vi "SMO.Control Experiment.getKHShuntType.vi"(8 "error in (no error)":errorcluster, 10 "getKHShuntType":T1, 11 "Control Experiment":refnum<class "SMO.Control Experiment.lvclass">) -> (0 "error out":errorcluster, 3 "Control Experiment out":refnum<class "SMO.Control Experiment.lvclass">)   [LabVIEW 2019, in "SMO.Control Experiment.lvclass"]
doc: "---------------------------------------------------------------\nJKI State Machine Objects™\nhttp://jki.net/state-machine-objects/\nCopyright (C) 2005-2015, JKI <info@jki.net>\nALL RIGHTS RESERVEDJKI State Machine Objects (SMO) 1.0.0.4\nJKI - JKI\nCopyright (c) 2015, JKI"
uses:
  SMO.Control Experiment.lvclass
  Typedefs/PublicEvents--SMO.Control Experiment.getKHShuntType.ctl
  SMO.Control Experiment.lvclass/SMO.Control Experiment.ctl
panel:
  # "For instructions on how to use the JKI State Machine Objects, examples and video tutorials, visit:\nhttp://jki.net/state-machine-objects/\n\nJKI State Machine Objects™\nhttp://jki.net/state-machine-objects/\nCopyright (C) 2005-2015, JKI <info@jki.net>\nALL RIGHTS RESERVED"
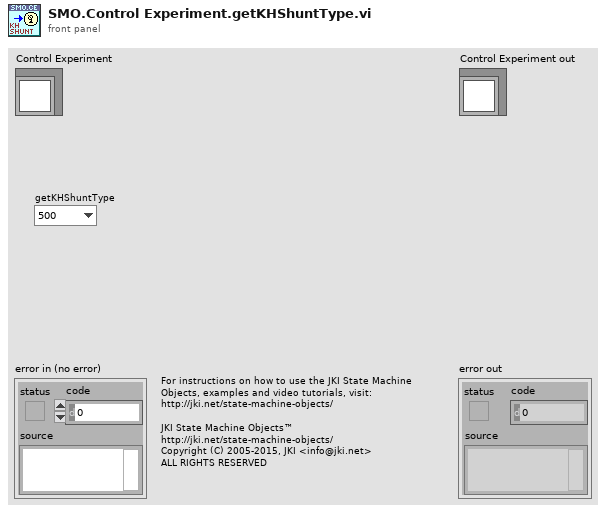
[diagram p1: front panel]
types:
  T1 = typedef "SMO.Control Experiment.lvclass/PublicEvents--SMO.Control Experiment.getKHShuntType.ctl" = enum16{"500", "10M"}
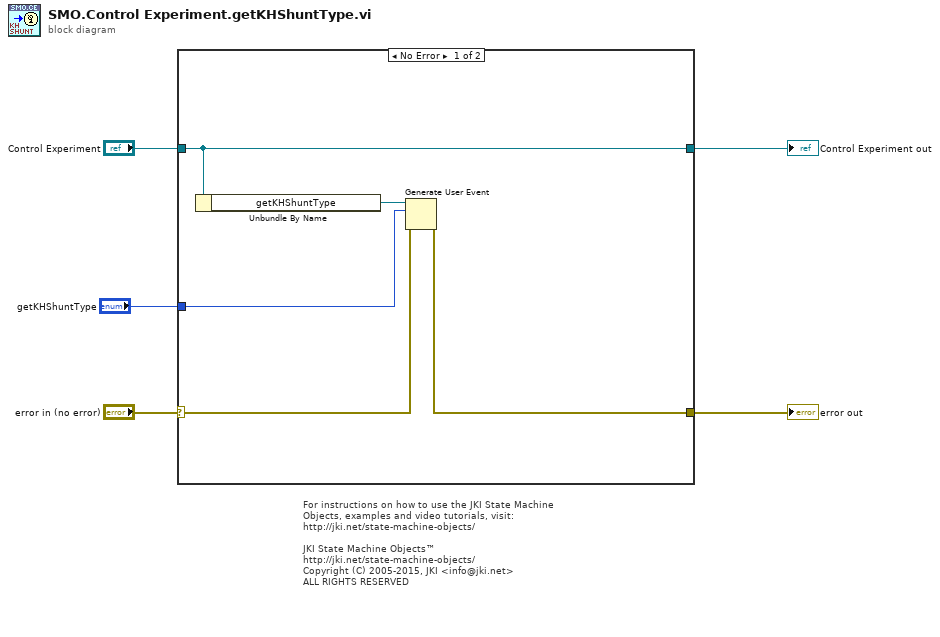
[diagram p0: block diagram]
diagram:
  # "For instructions on how to use the JKI State Machine Objects, examples and video tutorials, visit:\nhttp://jki.net/state-machine-objects/\n\nJKI State Machine Objects™\nhttp://jki.net/state-machine-objects/\nCopyright (C) 2005-2015, JKI <info@jki.net>\nALL RIGHTS RESERVED"
  n1 = case shown="No Error" "error in (no error)" {
    selector: "error in (no error)" -> [w10 w12]
    tunnel: [w8 w12] -> w4
    tunnel: [w7 w11] -> w5
    tunnel: "Control Experiment" -> [w7 w11]
    tunnel: "getKHShuntType" -> [w6 _]
    frame No Error {
      n2 = Unbundle By Name(w7) -> ("getKHShuntType"=w9:refnum<user-event>)
      n3 = Generate User Event(user event=w9, event data cluster=w6, error in=w10) -> (error out=w8:errorcluster)  [unwired: 1 in, 1 out]
    }
    frame Error {
    }
  }
  "error out" <- w4
  "Control Experiment out" <- w5
